vi "identify classes in memory.vi"(8 "error in":errorcluster, 10 "class cache data in":T1, 11 "Path":path) -> (0 "error out":errorcluster, 2 "class cache data out":T1)   [LabVIEW 2013, in "PL_class cache.lvlib"]
uses:
  PL_class cache.lvlib
  cached class information.ctl
  target class metadata.ctl
  class metadata.ctl
  <vilib>/NI/Tag Bus Module Framework/root configuration/Target Types.ctl
  Configuration Editor/Classes/Targets/Targets.lvclass
  Configuration Editor/Classes/Engine Parent/Engine Parent Editor Node.lvclass
  <vilib>/NI/Tag Bus Module Framework/root configuration/TBM configuration.lvclass
  <vilib>/NI/Configuration Framework/serializable configuration/NISE_CEF_serializable configuration.lvclass
  Configuration Editor/Classes/Module editor node/module editor node.lvclass
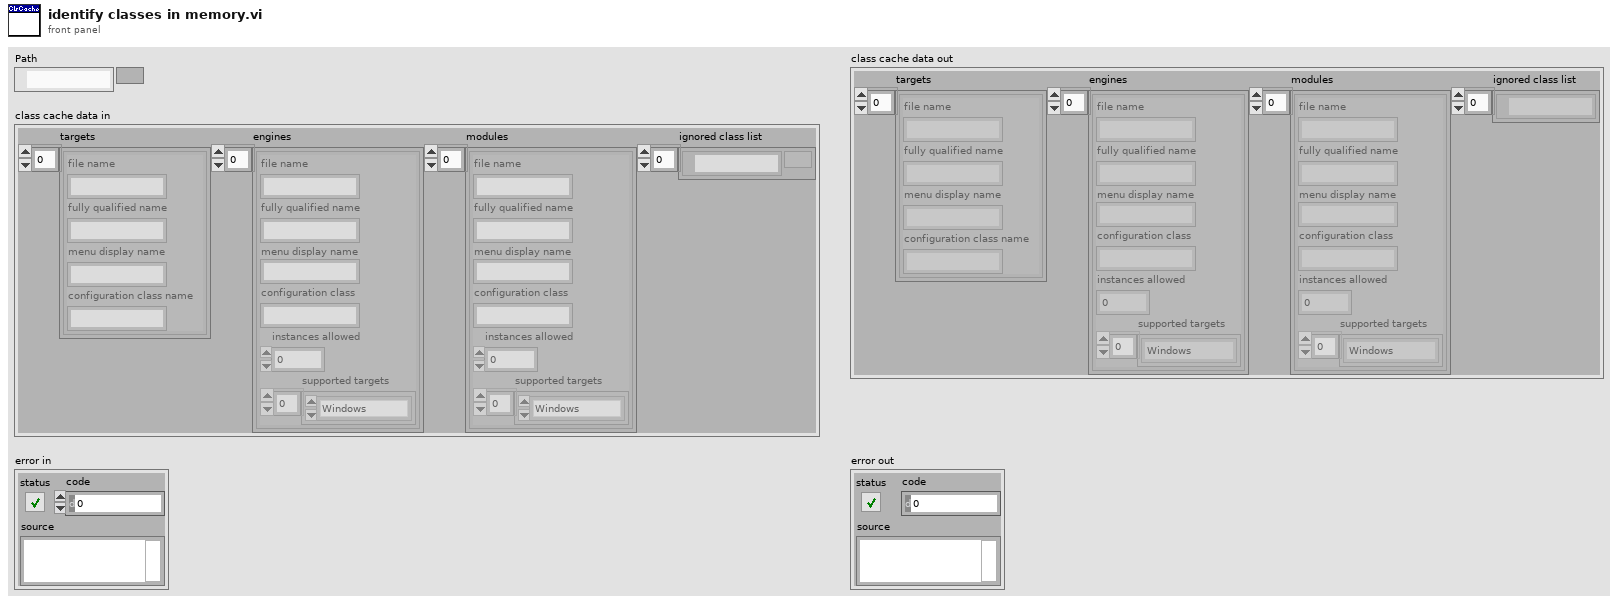
[diagram p1: front panel]
types:
  T1 = typedef "PL_class cache.lvlib/cached class information.ctl" = cluster{"targets":T2[], "engines":T3[], "modules":T3[], "ignored class list":path[]}
  T2 = typedef "PL_class cache.lvlib/target class metadata.ctl" = cluster{"file name":string, "fully qualified name":string, "menu display name":string, "configuration class name":string}
  T3 = typedef "PL_class cache.lvlib/class metadata.ctl" = cluster{"file name":string, "fully qualified name":string, "menu display name":string, "configuration class":string, "instances allowed":i32, "supported targets":T4[]}
  T4 = typedef "TBM configuration.lvclass/Target Types.ctl" = enum16{"Windows", "Mac", "Linux", "Linux RT ARM", "VxWorks", "Pharlap", "Other", "Linux RT x64"}
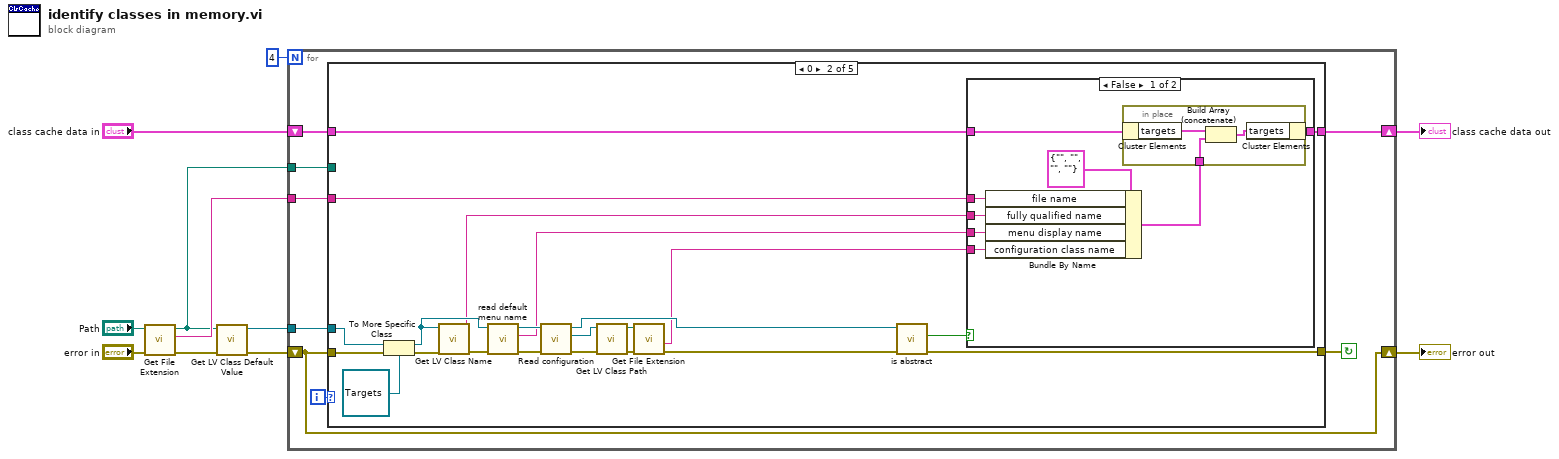
[diagram p0: block diagram]
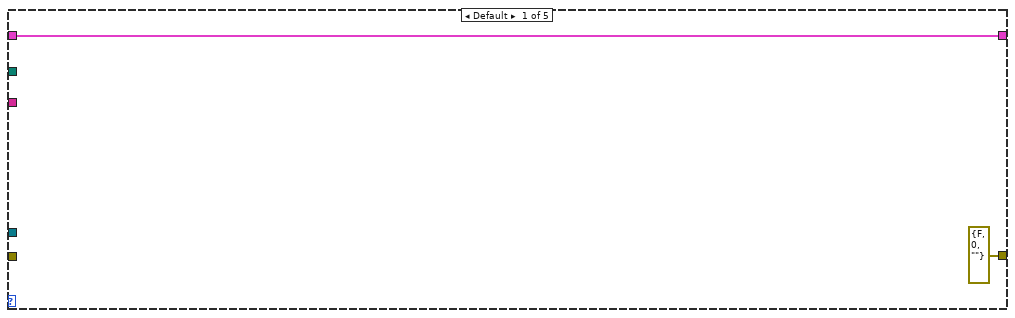
[diagram p2: hidden frame]
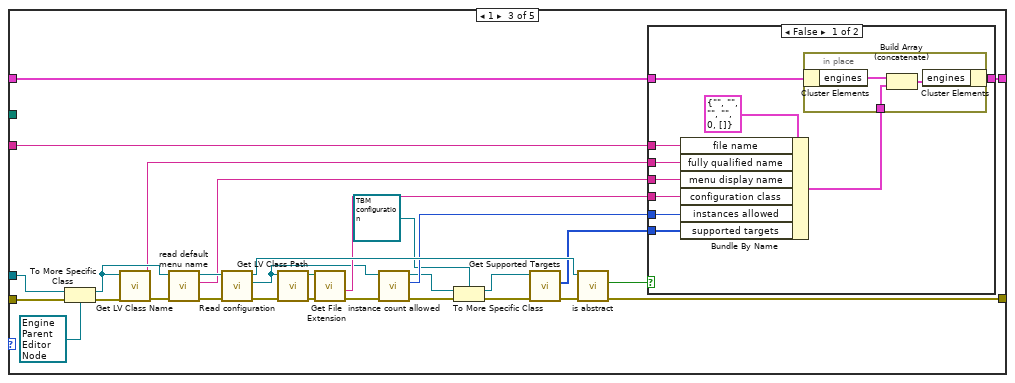
[diagram p4: hidden frame]
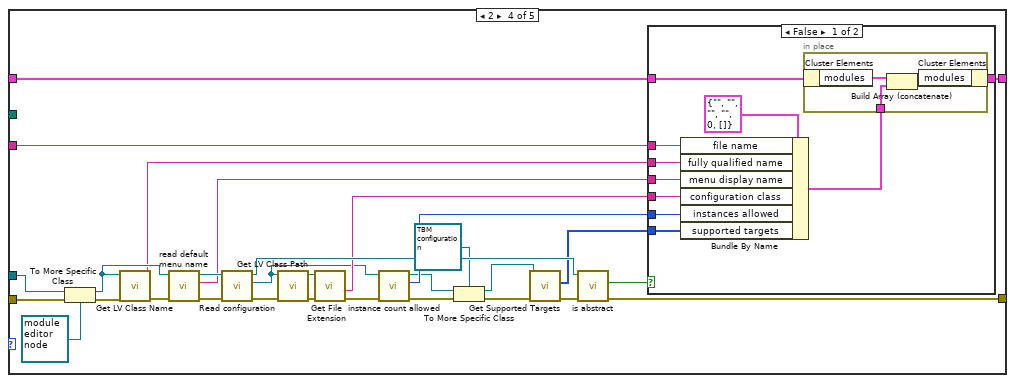
[diagram p6: hidden frame]
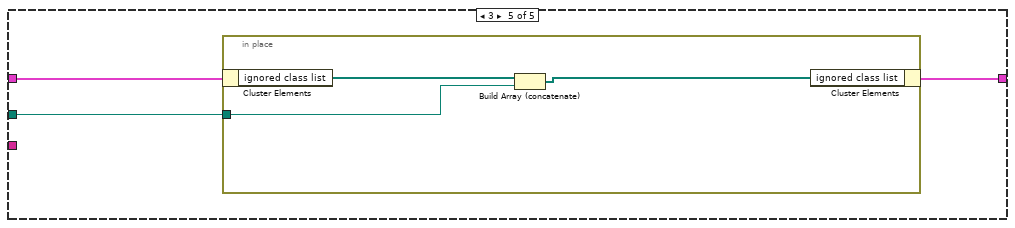
[diagram p8: hidden frame]
diagram:
  n1 = call <vilib>:"Get File Extension.vi"("error in (no error)"="error in", "file"="Path") -> ("error out"=w10:errorcluster, "lowercase file extension"=w6:string, "dup file"=w1:path)  [unwired: 6 in, 1 out]
  n2 = call <vilib>:"Get LV Class Default Value.vi"("error in (no error)"=w10, "class path"=w1) -> ("error out"=w8:errorcluster, "object"=w7:refnum<class>)  [unwired: 8 in]
  n3 = for {
    N: 4 -> [_]
    shift-right: [w16] -> w2
    shift-left: w8 -> [w16]
    tunnel: w7 -> [w15]
    tunnel: w6 -> [w13]
    shift-right: [w17] -> w3
    shift-left: "class cache data in" -> [w18]
    tunnel: w1 -> [w12]
    i -> [w19]
    stop <- w14 continue-if-true
    n4 = case shown="0" w19 {
      tunnel: w18 -> [w21 w28 w72 w116 w146]
      tunnel: [w21 w27 w71 w115 w145] -> w17
      tunnel: w16 -> [_ w43 w85 w129 _]
      tunnel: w15 -> [_ w42 w84 w128 _]
      tunnel: [errorcluster {"status"=FALSE, "code"=0, "source"=""} ("error out") w29 w73 w117 _] -> w14
      tunnel: w13 -> [_ w25 w69 w113 _]
      tunnel: w12 -> [_ _ _ _ w144]
      frame Default {
      }
      frame 0 {
        n5 = To More Specific Class(target class=refnum<class "Targets.lvclass"> refnum ("Targets"), reference=w42, error in=w43) -> (specific class reference=w30:refnum<class "Targets.lvclass">, error out=w40:errorcluster)
        n6 = call <vilib>:"Get LV Class Name.vi"("error in (no error)"=w40, "object"=w30) -> ("error out"=w31:errorcluster, "class name"=w26:string)  [unwired: 8 in]
        n7 = call-dynamic "read default menu name.vi"("error in"=w31, "Targets in"=w30) -> ("error out"=w38:errorcluster, "default menu name"=w24:string, "Targets out"=w39:refnum<class "Targets.lvclass">)  [unwired: 7 in]
        n8 = call-dynamic "Read configuration.vi"("error in"=w38, "NISE_CEF_serializable node in"=w39) -> ("error out"=w34:errorcluster, "configuration"=w33:refnum<class "NISE_CEF_serializable configuration.lvclass">, "NISE_CEF_serializable node out"=w36:refnum<class "Targets.lvclass">)  [unwired: 7 in]
        n9 = call <vilib>:"Get LV Class Path.vi"("error in (no error)"=w34, "object"=w33) -> ("error out"=w35:errorcluster, "class path"=w32:path)  [unwired: 8 in]
        n10 = call <vilib>:"Get File Extension.vi"("error in (no error)"=w35, "file"=w32) -> ("error out"=w37:errorcluster, "filename without extension"=w23:string)  [unwired: 6 in, 2 out]
        n11 = call-dynamic "is abstract.vi"("error in"=w37, "Targets in"=w36) -> ("error out"=w29:errorcluster, "abstract"=w22:bool)  [unwired: 7 in, 1 out]
        n12 = case shown="False" w22 {
          tunnel: w28 -> [w49 w55]
          tunnel: [w48 w55] -> w27
          tunnel: w26 -> [w47 _]
          tunnel: w25 -> [w46 _]
          tunnel: w24 -> [w45 _]
          tunnel: w23 -> [w44 _]
          frame False {
            n13 = Bundle By Name(cluster=T2 {"file name"="", "fully qualified name"="", "menu display name"="", "configuration class name"=""} ("class metadata"), "file name"=w46, "fully qualified name"=w47, "menu display name"=w45, "configuration class name"=w44) -> (w50:T2)
            n14 = in-place {
              in-place-border: w50 -> [w52]
              n15 = in-place-cluster #1(w49) -> ("targets"=w54:T2[])
              n16 = Build Array (concatenate)(w54, w52) -> (w53:T2[])
              n17 = in-place-cluster #1("targets"=w53) -> (w48:T1)
            }
          }
          frame True {
          }
        }
      }
      frame 1 {
        n18 = To More Specific Class(target class=refnum<class "Engine Parent Editor Node.lvclass"> refnum ("Engine Parent.lvclass"), reference=w84, error in=w85) -> (specific class reference=w74:refnum<class "Engine Parent Editor Node.lvclass">, error out=w83:errorcluster)
        n19 = call <vilib>:"Get LV Class Name.vi"("error in (no error)"=w83, "object"=w74) -> ("error out"=w75:errorcluster, "class name"=w70:string)  [unwired: 8 in]
        n20 = call-dynamic "read default menu name.vi"("error in"=w75, "Engine Parent Editor Node in"=w74) -> ("error out"=w81:errorcluster, "default menu name"=w68:string, "Engine Parent Editor Node out"=w82:refnum<class "Engine Parent Editor Node.lvclass">)  [unwired: 7 in]
        n21 = call-dynamic "Read configuration.vi"("error in"=w81, "NISE_CEF_serializable node in"=w82) -> ("error out"=w77:errorcluster, "configuration"=w63:refnum<class "NISE_CEF_serializable configuration.lvclass">, "NISE_CEF_serializable node out"=w79:refnum<class "Engine Parent Editor Node.lvclass">)  [unwired: 7 in]
        n22 = call <vilib>:"Get LV Class Path.vi"("error in (no error)"=w77, "object"=w63) -> ("error out"=w78:errorcluster, "class path"=w76:path)  [unwired: 8 in]
        n23 = call <vilib>:"Get File Extension.vi"("error in (no error)"=w78, "file"=w76) -> ("error out"=w80:errorcluster, "filename without extension"=w67:string)  [unwired: 6 in, 2 out]
        n24 = call-dynamic "instance count allowed.vi"("error in"=w80, "configuration in"=w63) -> ("error out"=w64:errorcluster, "instances allowed"=w61:i32, "configuration out"=w56:refnum<class "NISE_CEF_serializable configuration.lvclass">)  [unwired: 7 in]
        n25 = To More Specific Class(target class=refnum<class "TBM configuration.lvclass"> refnum ("configuration in"), reference=w56, error in=w64) -> (specific class reference=w58:refnum<class "TBM configuration.lvclass">, error out=w59:errorcluster)
        n26 = call-dynamic "Get Supported Targets.vi"("error in"=w59, "configuration in"=w58) -> ("error out"=w62:errorcluster, "supported targets"=w60:T4[])  [unwired: 7 in, 1 out]
        n27 = call-dynamic "is abstract.vi"("error in"=w62, "Engine Parent Editor Node in"=w79) -> ("error out"=w73:errorcluster, "abstract"=w66:bool)  [unwired: 7 in, 1 out]
        n28 = case shown="False" w66 {
          tunnel: w72 -> [w94 w99]
          tunnel: [w93 w99] -> w71
          tunnel: w70 -> [w92 _]
          tunnel: w69 -> [w91 _]
          tunnel: w68 -> [w90 _]
          tunnel: w67 -> [w89 _]
          tunnel: w61 -> [w87 _]
          tunnel: w60 -> [w86 _]
          frame False {
            n29 = Bundle By Name(cluster=T3 {"file name"="", "fully qualified name"="", "menu display name"="", "configuration class"="", "instances allowed"=0, "supported targets"=[]} ("class metadata"), "file name"=w91, "fully qualified name"=w92, "menu display name"=w90, "configuration class"=w89, "instances allowed"=w87, "supported targets"=w86) -> (w95:T3)
            n30 = in-place {
              in-place-border: w95 -> [w96]
              n31 = in-place-cluster #2(w94) -> ("engines"=w98:T3[])
              n32 = Build Array (concatenate)(w98, w96) -> (w97:T3[])
              n33 = in-place-cluster #2("engines"=w97) -> (w93:T1)
            }
          }
          frame True {
          }
        }
      }
      frame 2 {
        n34 = To More Specific Class(target class=refnum<class "module editor node.lvclass"> refnum ("Component Parent.lvclass"), reference=w128, error in=w129) -> (specific class reference=w118:refnum<class "module editor node.lvclass">, error out=w127:errorcluster)
        n35 = call <vilib>:"Get LV Class Name.vi"("error in (no error)"=w127, "object"=w118) -> ("error out"=w119:errorcluster, "class name"=w114:string)  [unwired: 8 in]
        n36 = call-dynamic "read default menu name.vi"("error in"=w119, "module editor node in"=w118) -> ("error out"=w125:errorcluster, "default menu name"=w112:string, "module editor node out"=w126:refnum<class "module editor node.lvclass">)  [unwired: 7 in]
        n37 = call-dynamic "Read configuration.vi"("error in"=w125, "NISE_CEF_serializable node in"=w126) -> ("error out"=w121:errorcluster, "configuration"=w108:refnum<class "NISE_CEF_serializable configuration.lvclass">, "NISE_CEF_serializable node out"=w123:refnum<class "module editor node.lvclass">)  [unwired: 7 in]
        n38 = call <vilib>:"Get LV Class Path.vi"("error in (no error)"=w121, "object"=w108) -> ("error out"=w122:errorcluster, "class path"=w120:path)  [unwired: 8 in]
        n39 = call <vilib>:"Get File Extension.vi"("error in (no error)"=w122, "file"=w120) -> ("error out"=w124:errorcluster, "filename without extension"=w111:string)  [unwired: 6 in, 2 out]
        n40 = call-dynamic "instance count allowed.vi"("error in"=w124, "configuration in"=w108) -> ("error out"=w109:errorcluster, "instances allowed"=w106:i32, "configuration out"=w102:refnum<class "NISE_CEF_serializable configuration.lvclass">)  [unwired: 7 in]
        n41 = To More Specific Class(target class=refnum<class "TBM configuration.lvclass"> refnum ("configuration in"), reference=w102, error in=w109) -> (specific class reference=w100:refnum<class "TBM configuration.lvclass">, error out=w103:errorcluster)
        n42 = call-dynamic "Get Supported Targets.vi"("error in"=w103, "configuration in"=w100) -> ("error out"=w107:errorcluster, "supported targets"=w105:T4[])  [unwired: 7 in, 1 out]
        n43 = call-dynamic "is abstract.vi"("error in"=w107, "module editor node in"=w123) -> ("error out"=w117:errorcluster, "abstract"=w110:bool)  [unwired: 7 in, 1 out]
        n44 = case shown="False" w110 {
          tunnel: w116 -> [w138 w143]
          tunnel: [w137 w143] -> w115
          tunnel: w114 -> [w136 _]
          tunnel: w113 -> [w135 _]
          tunnel: w112 -> [w134 _]
          tunnel: w111 -> [w133 _]
          tunnel: w106 -> [w131 _]
          tunnel: w105 -> [w130 _]
          frame False {
            n45 = Bundle By Name(cluster=T3 {"file name"="", "fully qualified name"="", "menu display name"="", "configuration class"="", "instances allowed"=0, "supported targets"=[]} ("class metadata"), "file name"=w135, "fully qualified name"=w136, "menu display name"=w134, "configuration class"=w133, "instances allowed"=w131, "supported targets"=w130) -> (w139:T3)
            n46 = in-place {
              in-place-border: w139 -> [w140]
              n47 = in-place-cluster #3(w138) -> ("modules"=w142:T3[])
              n48 = Build Array (concatenate)(w142, w140) -> (w141:T3[])
              n49 = in-place-cluster #3("modules"=w141) -> (w137:T1)
            }
          }
          frame True {
          }
        }
      }
      frame 3 {
        n50 = in-place {
          in-place-border: w144 -> [w147]
          n51 = in-place-cluster #4(w146) -> ("ignored class list"=w149:path[])
          n52 = Build Array (concatenate)(w149, w147) -> (w148:path[])
          n53 = in-place-cluster #4("ignored class list"=w148) -> (w145:T1)
        }
      }
    }
  }
  "class cache data out" <- w3
  "error out" <- w2
